vi "GlobalDataNum.vi"() -> ()   [LabVIEW 2015]
panel:
  out "DataNum":dbl[](array[numeric])
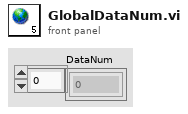
[diagram p1: front panel]
diagram:
